vi "esP32DataToInfo.vi"(7 "Enc_values_in":T1, 8 "error in":errorcluster, 10 "Cluster_modbus":T5, 11 "new_data?":bool) -> (0 "error out":errorcluster, 5 "Enc_values_out":T1)   [LabVIEW 2026]
uses:
  Control/Ctrl_Modbus28.ctl
  Control/Ctr_Enc_Values.ctl
  Control/Ctrl_datos6motores_final.ctl
  Control/Ctrl_Motores_Valores.ctl
  Control/Ctrl_Errores.ctl
  Ctrl_MainPanelGui.ctl
  <vilib>/ptbypt/NI_PtbyPt.lvlib
  Ctrl_EstadosMotor.ctl
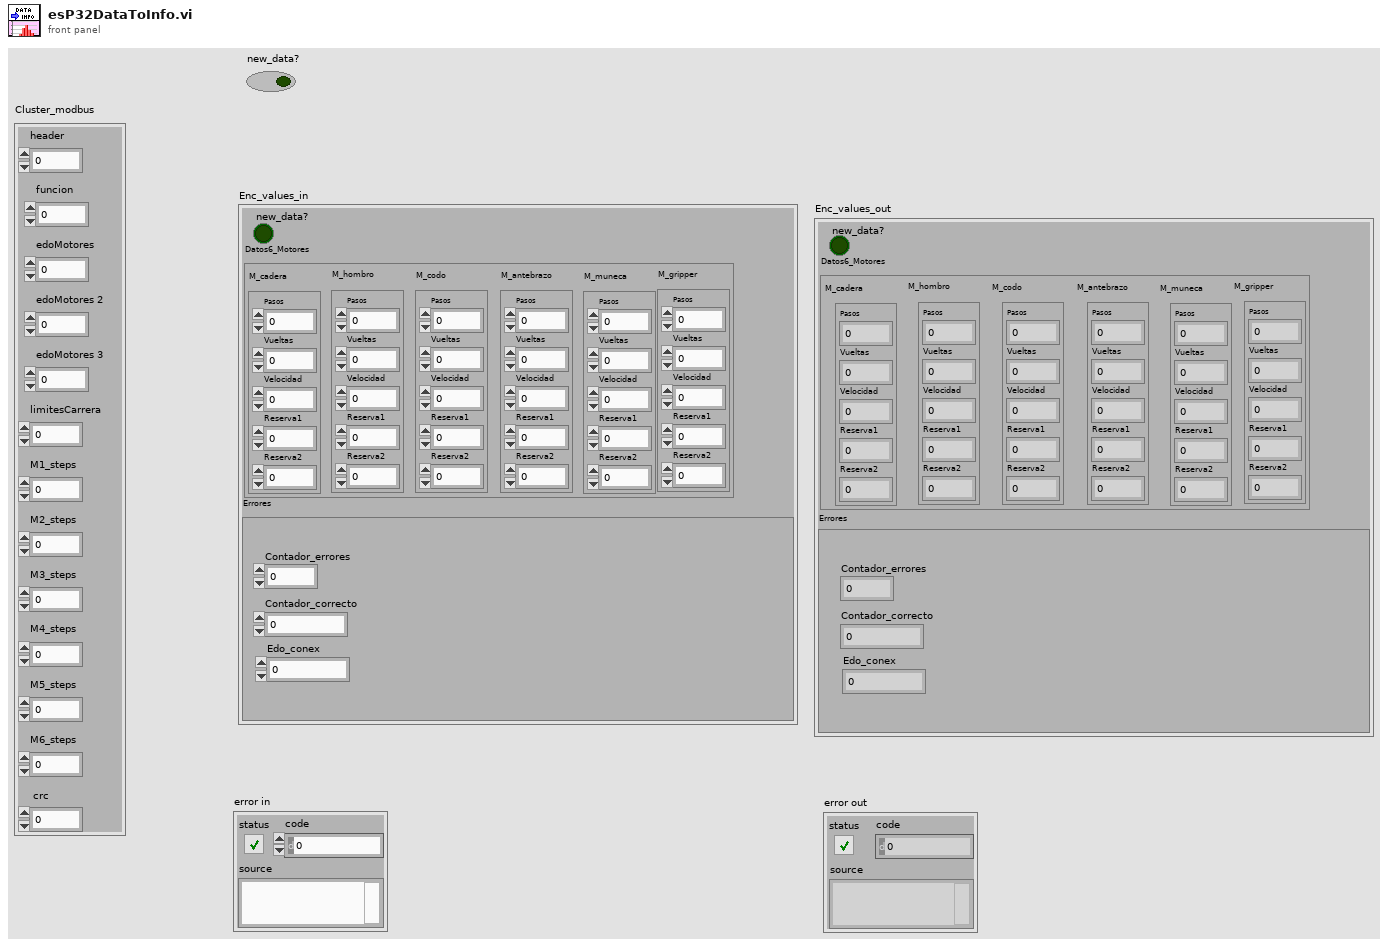
[diagram p1: front panel]
types:
  T1 = typedef "Ctr_Enc_Values.ctl" = cluster{"Datos6_Motores":T2, "Errores":T4, "new_data?":bool}
  T2 = typedef "Ctrl_datos6motores_final.ctl" = cluster{"M_cadera":T3, "M_hombro":T3, "M_codo":T3, "M_antebrazo":T3, "M_muneca":T3, "M_gripper":T3}
  T3 = typedef "Ctrl_Motores_Valores.ctl" = cluster{"Pasos":i32, "Vueltas":i16, "Velocidad":dbl, "Reserva1":u8, "Reserva2":u8}
  T4 = typedef "Ctrl_Errores.ctl" = cluster{"Contador_correcto":u32, "Contador_errores":u32, "Edo_conex":u32}
  T5 = typedef "Ctrl_Modbus28.ctl" = cluster{"header":u8, "funcion":u8, "edoMotores":u8, "edoMotores 2":u8, "edoMotores 3":u8, "limitesCarrera":u8, "M1_steps":i32, "M2_steps":i32, "M3_steps":i32, "M4_steps":i32, "M5_steps":i32, "M6_steps":i32, " crc":u8}
  T6 = typedef "Ctrl_EstadosMotor.ctl" = enum16{"SET_DATA", "GET_DATA", "START"}
  T7 = typedef "Ctrl_MainPanelGui.ctl" = enum16{"Start", "SET_DATA", "GET_DATA", "STOP"}
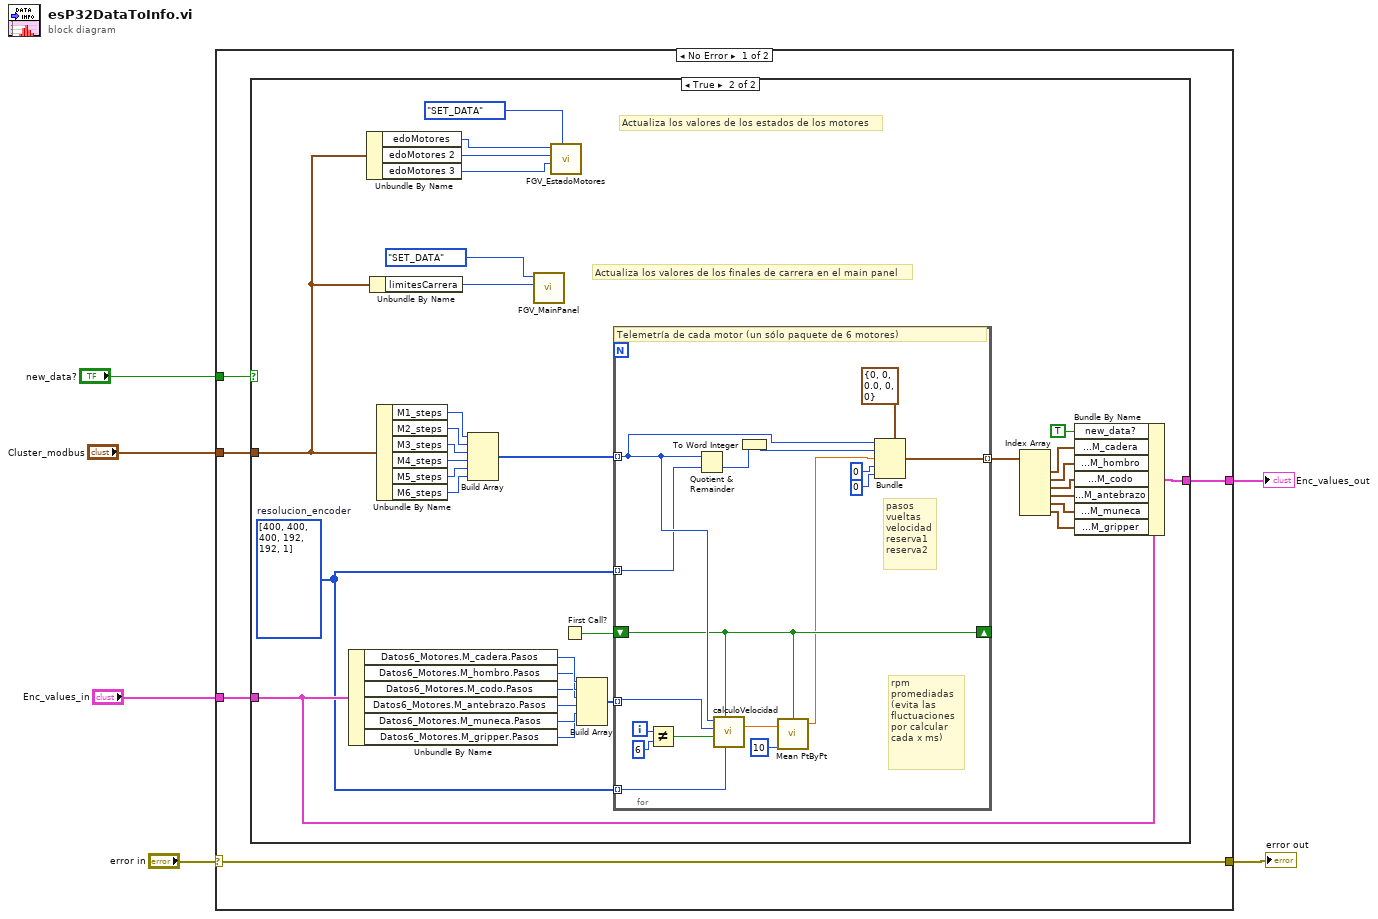
[diagram p0: block diagram]
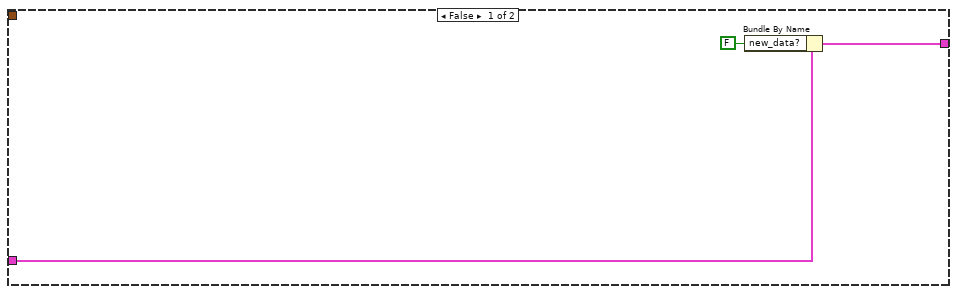
[diagram p2: hidden frame]
diagram:
  n1 = case shown="No Error" "error in" {
    selector: "error in" -> [w11 w66]
    tunnel: [w11 w66] -> w5
    tunnel: "Cluster_modbus" -> [w10 _]
    tunnel: "new_data?" -> [w9 _]
    tunnel: "Enc_values_in" -> [w8 w65]
    tunnel: [w7 w65] -> w1
    frame No Error {
      n2 = case shown="True" w9 {
        tunnel: w10 -> [_ w19]
        tunnel: w8 -> [w13 w32]
        tunnel: [w14 w25] -> w7
        frame False {
          n3 = Bundle By Name(cluster=w13, "new_data?"=FALSE) -> (w14:T1)
        }
        frame True {
          w23 = i32[] [400, 400, 400, 192, 192, 1]  # resolucion_encoder
          # "Actualiza los valores de los estados de los motores"
          # "Actualiza los valores de los finales de carrera en el main panel"
          n4 = Unbundle By Name(w32) -> ("Datos6_Motores.M_cadera.Pasos"=w40:i32, "Datos6_Motores.M_hombro.Pasos"=w39:i32, "Datos6_Motores.M_codo.Pasos"=w38:i32, "Datos6_Motores.M_antebrazo.Pasos"=w37:i32, "Datos6_Motores.M_muneca.Pasos"=w36:i32, "Datos6_Motores.M_gripper.Pasos"=w35:i32)
          n5 = Unbundle By Name(w19) -> ("edoMotores"=w18:u8, "edoMotores 2"=w17:u8, "edoMotores 3"=w16:u8)
          n6 = Unbundle By Name(w19) -> ("limitesCarrera"=w21:u8)
          n7 = Unbundle By Name(w19) -> ("M1_steps"=w47:i32, "M2_steps"=w46:i32, "M3_steps"=w45:i32, "M4_steps"=w44:i32, "M5_steps"=w43:i32, "M6_steps"=w42:i32)
          n8 = Build Array(w47, w46, w45, w44, w43, w42) -> (w41:i32[])
          n9 = call "FGV_MainPanel.vi"("LS_U8"=w21, "Estado"=Ctrl_MainPanelGui."SET_DATA") -> ()  [unwired: 8 in, 2 out]
          n10 = call "FGV_EstadoMotores.vi"("Control"=Ctrl_EstadosMotor."SET_DATA", "edoMotores3_in"=w16, "edoMotores2_in"=w17, "edoMotores_in"=w18) -> ()  [unwired: 7 in, 1 out]
          n11 = First Call?() -> (First Call?: T/F=w22:bool)
          n12 = Build Array(w40, w39, w38, w37, w36, w35) -> (w34:i32[])
          n13 = for {
            tunnel: w41 -> [w60] mode=indexing
            tunnel: w23 -> [w56] mode=indexing
            tunnel: w34 -> [w63] mode=indexing
            tunnel: [w62] -> w33 mode=indexing
            tunnel: w23 -> [w55] mode=indexing
            shift-right: [w50] -> _
            shift-left: w22 -> [w50]
            i -> [w54]
            # "rpm promediadas\n(evita las fluctuaciones por calcular cada x ms)"
            # "pasos\nvueltas\nvelocidad\nreserva1\nreserva2"
            # "Telemetría de cada motor (un sólo paquete de 6 motores)"
            n14 = Not Equal?(x=w54, y=6) -> (x != y?=w51:bool)
            n15 = Quotient & Remainder(x=w60, y=w56) -> (floor(x/y)=w64:i32)  [unwired: 1 out]
            n16 = call "calculoVelocidad.vi"("Resolucion"=w55, "primera_iteracion?"=w50, "motor_gripper?"=w51, "Pasos_anteriores"=w63, "Pasos_nuevos"=w60) -> ("RPM"=w49:dbl)  [unwired: 6 in]
            n17 = To Word Integer(number=w64) -> (16bit integer=w59:i16)
            n18 = call <vilib>:"Mean PtByPt.vi"("x"=w49, "sample length"=10, "initialize"=w50) -> ("mean"=w48:dbl)  [unwired: 1 in, 1 out]
            n19 = Bundle(cluster=T3 {"Pasos"=0, "Vueltas"=0, "Velocidad"=0.0, "Reserva1"=0, "Reserva2"=0} ("M_gripper"), "Pasos"=w60, "Vueltas"=w59, "Velocidad"=w48, "Reserva1"=u8 0, "Reserva2"=u8 0) -> (w62:T3)
          }
          n20 = Index Array(array=w33) -> (element #1=w31:T3, element #2=w30:T3, element #3=w29:T3, element #4=w28:T3, element #5=w27:T3, element #6=w26:T3)  [unwired: 6 in]
          n21 = Bundle By Name(cluster=w32, "new_data?"=TRUE, "Datos6_Motores.M_cadera"=w31, "Datos6_Motores.M_hombro"=w30, "Datos6_Motores.M_codo"=w29, "Datos6_Motores.M_antebrazo"=w28, "Datos6_Motores.M_muneca"=w27, "Datos6_Motores.M_gripper"=w26) -> (w25:T1)
        }
      }
    }
    frame Error {
    }
  }
  "error out" <- w5
  "Enc_values_out" <- w1
